vi "Get Scanner.vi"(8 "error in (no error)":errorcluster, 11 "Spectrometer Triax 550 in":refnum<class "Spectrometer Triax 550.lvclass">) -> (0 "error out":errorcluster, 2 "Default Scanner out":refnum<class "Scanner.lvclass">)   [LabVIEW 2017, in "Spectrometer Triax 550.lvclass"]
doc: "(Dynamic) Returns the default Scanner object that scans over this Scannable. (Note that a Scannable may have multiple Scanners associated with it.) A Scanner is an analogue to an Iterator class in other languages."
uses:
  Spectrometer Triax 550.lvclass
  Scanners/Scanner/Scanner.lvclass
  Scanners/Wavelength/Wavelength.lvclass
  C:/LabVIEW-programs-dev/Scanners/Scanner/Scanner.lvclass
  Utility Classes/Scannable/Scannable.lvclass
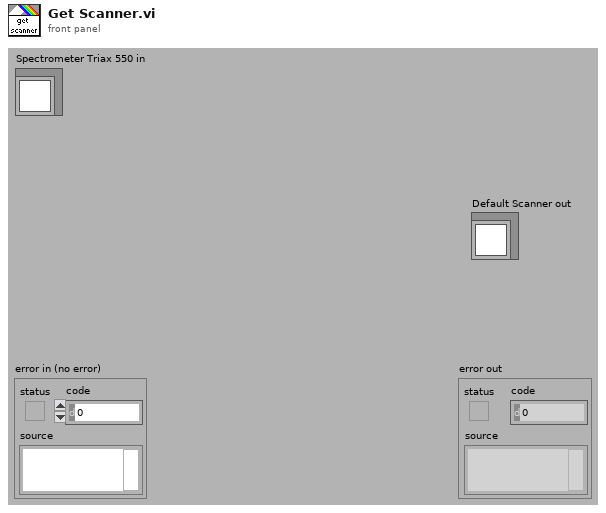
[diagram p1: front panel]
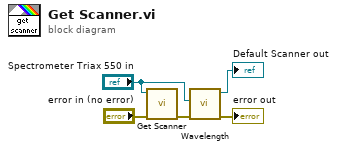
[diagram p0: block diagram]
diagram:
  n1 = call-parent "Get Scanner.vi"("error in (no error)"="error in (no error)", "Scannable in"="Spectrometer Triax 550 in") -> ("error out"=w1:errorcluster)  [unwired: 9 out]
  n2 = call "Wavelength.vi"("error in (no error)"=w1, "Spectrometer Triax 550.lvclass"="Spectrometer Triax 550 in") -> ("error out"=→"error out":errorcluster, "Wavelength out"=→"Default Scanner out":refnum<class "Wavelength.lvclass">)  [unwired: 8 out]
